vi "GDSProject_Create.vi"(1 "ProjectTreePosition(String or Project Item Ref)":variant, 2 "AllowPopUpDilaog(True)":bool=TRUE, 5 "error in (no error)":errorcluster) -> (14 "Project Refnum":refnum<vi>, 15 "Project Item":refnum<vi>, 17 "App":refnum<vi>, 19 "error out":errorcluster)   [LabVIEW 2016]
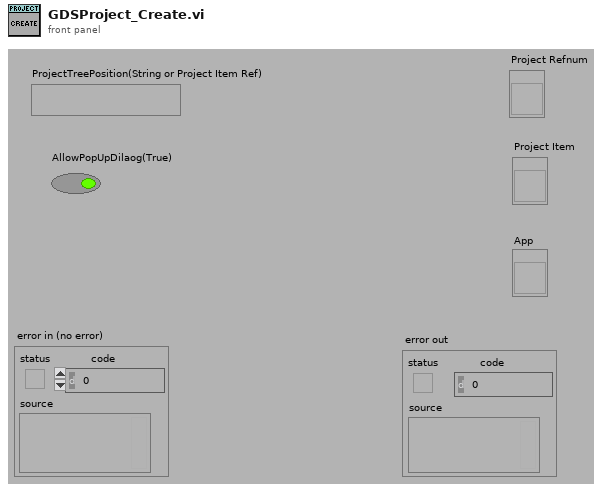
[diagram p1: front panel]
types:
  T1 = enum16{"Left Button", "Center Button", "Right Button", "Window Close"}
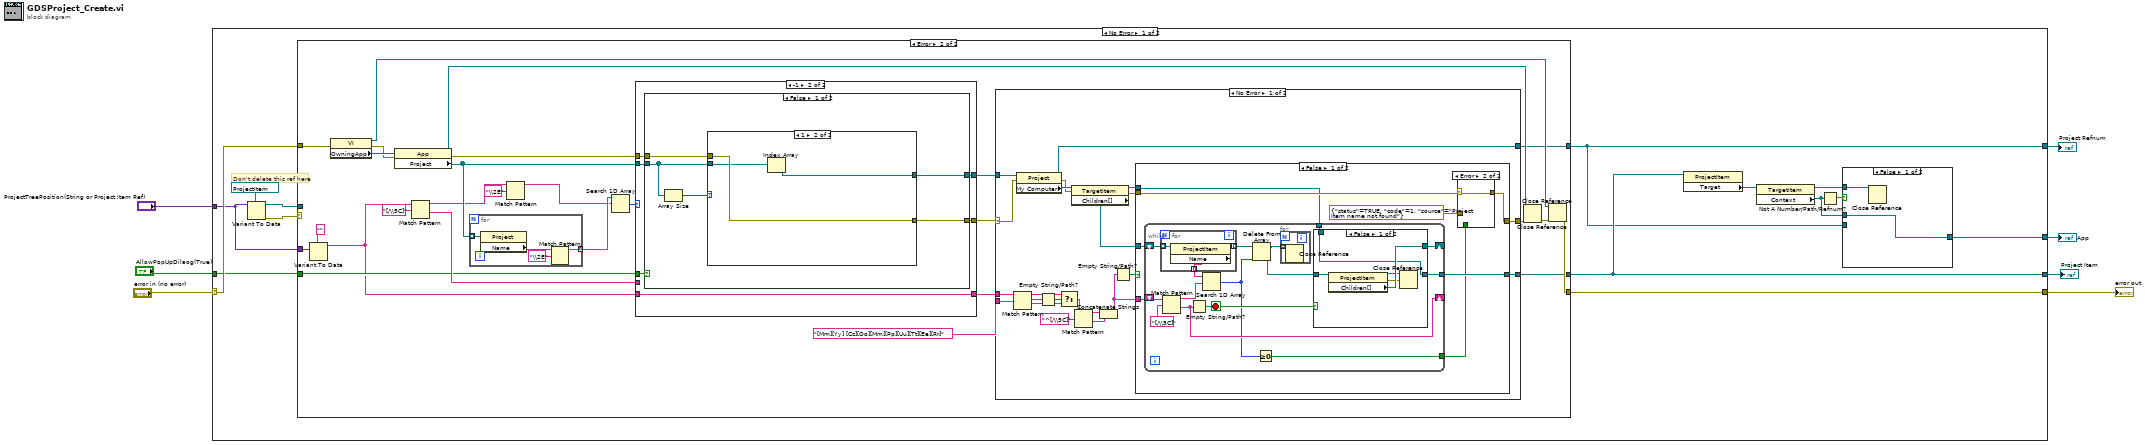
[diagram p0: block diagram]
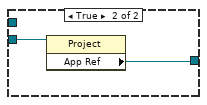
[diagram p2: hidden frame]
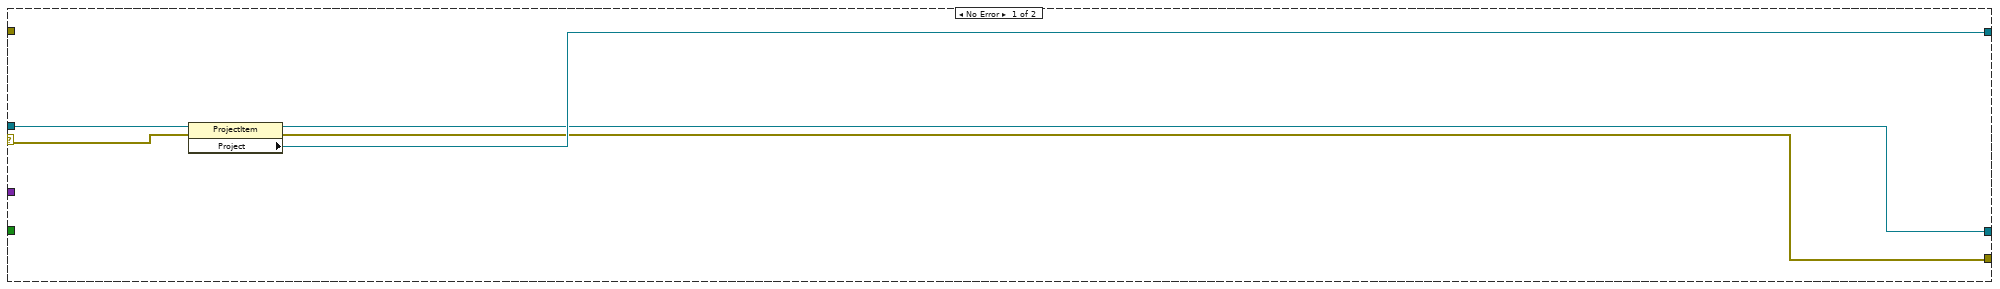
[diagram p3: hidden frame]
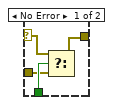
[diagram p4: hidden frame]
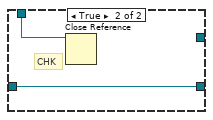
[diagram p5: hidden frame]
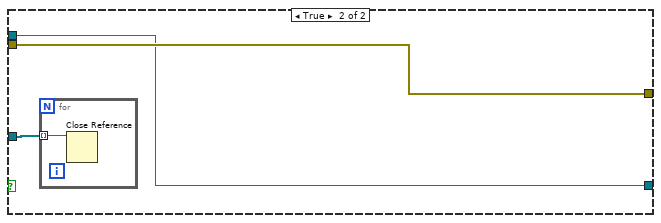
[diagram p6: hidden frame]
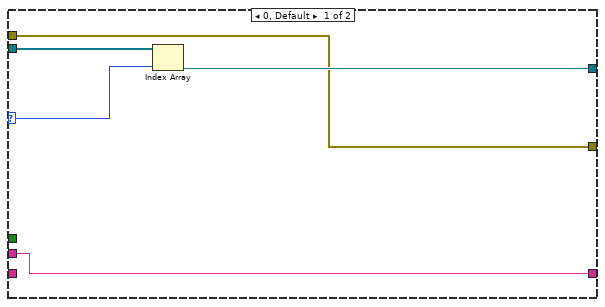
[diagram p8: hidden frame]
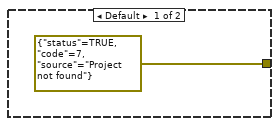
[diagram p9: hidden frame]
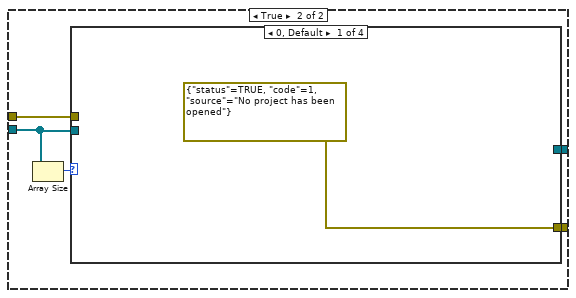
[diagram p10: hidden frame]
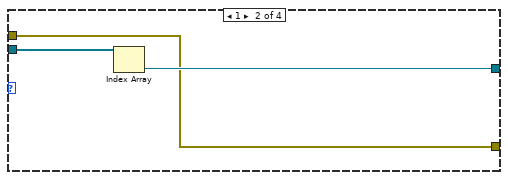
[diagram p11: hidden frame]
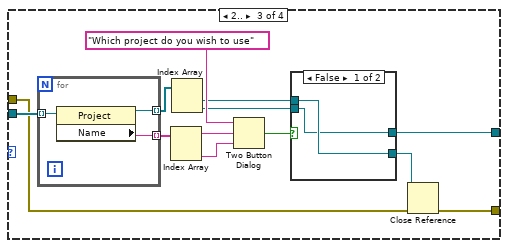
[diagram p12: hidden frame]
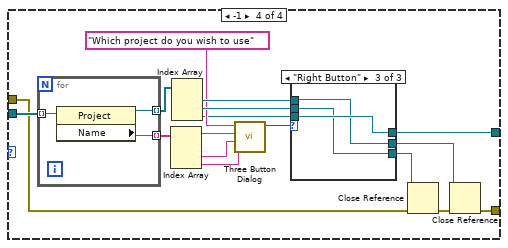
[diagram p14: hidden frame]
diagram:
  n1 = case shown="No Error" "error in (no error)" {
    selector: "error in (no error)" -> [w21 w206]
    tunnel: [w20 w206] -> w6
    tunnel: "ProjectTreePosition(String or Project Item Ref)" -> [w15 _]
    tunnel: [w11 _] -> w4
    tunnel: [w10 _] -> w3
    tunnel: "AllowPopUpDilaog(True)" -> [w19 _]
    tunnel: [w9 _] -> w1
    frame No Error {
      # "Don't delete this ref here"
      n2 = Variant To Data(type=refnum<vi> refnum ("Project Item"), Variant=w15) -> (data=w16:refnum<vi>, error out=w17:errorcluster)  [unwired: 1 in]
      n3 = case shown="Error" w17 {
        selector: w17 -> [w26 _]
        tunnel: w21 -> [_ w56]
        tunnel: [w29 w51] -> w20
        tunnel: [w28 w41] -> w11
        tunnel: [w30 w36] -> w10
        tunnel: w19 -> [_ w35]
        tunnel: w16 -> [w27 _]
        tunnel: w15 -> [_ w33]
        frame No Error {
          n4 = property class="ProjectItem"(reference=w27, error in=w26) -> (reference out=w28:refnum<vi>, error out=w29:errorcluster, "Project"=w30:refnum<vi>)
        }
        frame Error {
          n5 = Variant To Data(type="" ("regular expression"), Variant=w33) -> (data=w31:string)  [unwired: 1 in, 1 out]
          n6 = property class="VI"(error in=w56) -> (reference out=w50:refnum<vi>, error out=w55:errorcluster, "OwningApp"=w57:refnum<vi>)  [unwired: 1 in]
          n7 = property class="App"(reference=w57, error in=w55) -> (reference out=w53:refnum<vi>, error out=w54:errorcluster, "Project"=w49:refnum<vi>[])
          n8 = Match Pattern(string=w31, regular expression="[/\\5C]") -> (before substring=w38:string, after substring=w45:string)  [unwired: 1 in, 2 out]
          n9 = for {
            tunnel: w49 -> [w205] mode=indexing
            tunnel: [w202] -> w47 mode=indexing
            n10 = property class="Project"(reference=w205) -> ("Name"=w203:string)  [unwired: 1 in, 2 out]
            n11 = Match Pattern(string=w203, regular expression="\\2E") -> (before substring=w202:string)  [unwired: 1 in, 3 out]
          }
          n12 = Match Pattern(string=w38, regular expression="\\2E") -> (before substring=w37:string)  [unwired: 1 in, 3 out]
          n13 = Search 1D Array(1D array=w47, element=w37) -> (index of element=w46:i32)  [unwired: 1 in]
          n14 = case shown="-1" w46 {
            selector: w46 -> [w127 _]
            tunnel: [w126 w134] -> w44
            tunnel: w54 -> [w125 w133]
            tunnel: [w125 w132] -> w34
            tunnel: w49 -> [w128 w131]
            tunnel: w31 -> [_ w130]
            tunnel: w45 -> [w124 _]
            tunnel: [w124 w130] -> w43
            tunnel: w35 -> [_ w129]
            frame 0, Default {
              n15 = Index Array(array=w128, index=w127) -> (element=w126:refnum<vi>)
            }
            frame -1 {
              n16 = case shown="False" w129 {
                tunnel: [w135 w148] -> w134
                tunnel: w133 -> [w137 w146]
                tunnel: [w139 w145] -> w132
                tunnel: w131 -> [w136 w144]
                frame False {
                  n17 = Array Size(array=w136) -> (size(s)=w138:i32)
                  n18 = case shown="1" w138 {
                    tunnel: [errorcluster {"status"=TRUE, "code"=7, "source"="Project not found"} ("error out") w143] -> w139
                    tunnel: w137 -> [_ w143]
                    tunnel: w136 -> [_ w142]
                    tunnel: [_ w141] -> w135
                    frame Default {
                    }
                    frame 1 {
                      n19 = Index Array(array=w142) -> (element=w141:refnum<vi>)  [unwired: 1 in]
                    }
                  }
                }
                frame True {
                  n20 = Array Size(array=w144) -> (size(s)=w147:i32)
                  n21 = case shown="0, Default" w147 {
                    tunnel: w144 -> [_ w152 w165 w189]
                    tunnel: [_ w151 w157 w185] -> w148
                    tunnel: w146 -> [_ w150 w155 w183]
                    tunnel: [errorcluster {"status"=TRUE, "code"=1, "source"="No project has been opened"} ("error out") w150 w154 w175] -> w145
                    frame 0, Default {
                    }
                    frame 1 {
                      n22 = Index Array(array=w152) -> (element=w151:refnum<vi>)  [unwired: 1 in]
                    }
                    frame 2.. {
                      n23 = for {
                        tunnel: w165 -> [w172] mode=indexing
                        tunnel: [w171] -> w163 mode=indexing
                        tunnel: [w170] -> w160 mode=indexing
                        n24 = property class="Project"(reference=w172) -> (reference out=w170:refnum<vi>, "Name"=w171:string)  [unwired: 1 in, 1 out]
                      }
                      n25 = Index Array(array=w163) -> (element #1=w162:string, element #2=w161:string)  [unwired: 2 in]
                      n26 = Index Array(array=w160) -> (element #1=w158:refnum<vi>, element #2=w156:refnum<vi>)  [unwired: 2 in]
                      n27 = Two Button Dialog(message="Which project do you wish to use", 1:w161, 2:w162) -> (T button?=w159:bool)
                      n28 = case shown="False" w159 {
                        tunnel: w158 -> [w167 w169]
                        tunnel: [w166 w169] -> w157
                        tunnel: [w167 w168] -> w153
                        tunnel: w156 -> [w166 w168]
                        frame False {
                        }
                        frame True {
                        }
                      }
                      n29 = Close Reference(reference=w153, error in (no error)=w155) -> (error out=w154:errorcluster)
                    }
                    frame -1 {
                      n30 = for {
                        tunnel: w189 -> [w201] mode=indexing
                        tunnel: [w200] -> w188 mode=indexing
                        tunnel: [w199] -> w187 mode=indexing
                        n31 = property class="Project"(reference=w201) -> (reference out=w199:refnum<vi>, "Name"=w200:string)  [unwired: 1 in, 1 out]
                      }
                      n32 = Index Array(array=w188) -> (element #1=w180:string, element #2=w179:string, element #3=w178:string)  [unwired: 3 in]
                      n33 = Index Array(array=w187) -> (element #1=w186:refnum<vi>, element #2=w184:refnum<vi>, element #3=w174:refnum<vi>)  [unwired: 3 in]
                      n34 = call <vilib>:"Three Button Dialog.vi"("Right Button Text (\"Cancel\")"=w178, "Center Button Text (\"No\")"=w179, "Left Button Text (\"Yes\")"=w180, "message"="Which project do you wish to use") -> ("Which Button?"=w177:T1)  [unwired: 7 in]
                      n35 = case shown="\"Right Button\"" w177 {
                        tunnel: w186 -> [w192 w194 w197]
                        tunnel: [w192 w195 w198] -> w185
                        tunnel: [w191 w193 w196] -> w182
                        tunnel: w184 -> [w190 w195 w196]
                        tunnel: w174 -> [w191 w193 w198]
                        tunnel: [w190 w194 w197] -> w173
                        frame "Left Button", Default {
                        }
                        frame "Center Button" {
                        }
                        frame "Right Button" {
                        }
                      }
                      n36 = Close Reference(reference=w182, error in (no error)=w183) -> (error out=w176:errorcluster)
                      n37 = Close Reference(reference=w173, error in (no error)=w176) -> (error out=w175:errorcluster)
                    }
                  }
                }
              }
            }
          }
          n38 = case shown="No Error" w34 {
            selector: w34 -> [w59 w123]
            tunnel: w44 -> [w79 _]
            tunnel: w43 -> [w77 _]
            tunnel: "[Mm][Yy] [Cc][Oo][Mm][Pp][Uu][Tt][Ee][Rr]" ("regular expression") -> [w76 _]
            tunnel: [w70 _] -> w41
            tunnel: [w66 w123] -> w40
            tunnel: [w65 _] -> w36
            frame No Error {
              n39 = Match Pattern(string=w77, regular expression=w76) -> (before substring=w73:string, match substring=w75:string, after substring=w72:string)  [unwired: 1 in, 1 out]
              n40 = property class="Project"(reference=w79, error in=w59) -> (reference out=w65:refnum<vi>, error out=w69:errorcluster, "My Computer"=w78:refnum<vi>)
              n41 = Empty String/Path?(string/path=w75) -> (empty?=w74:bool)
              n42 = Select(t=w73, s=w74, f=w72) -> (s? t:f=w64:string)
              n43 = property class="TargetItem"(reference=w78, error in=w69) -> (reference out=w58:refnum<vi>, error out=w67:errorcluster, "Children[]"=w71:refnum<vi>[])
              n44 = Match Pattern(string=w64, regular expression="^[/\\5C]") -> (before substring=w62:string, after substring=w61:string)  [unwired: 1 in, 2 out]
              n45 = Concatenate Strings(w62, w61) -> (w60:string)
              n46 = Empty String/Path?(string/path=w60) -> (empty?=w68:bool)
              n47 = case shown="False" w68 {
                tunnel: w71 -> [w87 w119]
                tunnel: [w86 w120] -> w70
                tunnel: w60 -> [w85 _]
                tunnel: w67 -> [w84 w121]
                tunnel: [w82 w121] -> w66
                tunnel: w58 -> [w80 w120]
                frame False {
                  n48 = while {
                    shift-right: [w100] -> _
                    shift-left: w87 -> [w107]
                    tunnel: [w99] -> w86
                    shift-right: [w97] -> _
                    shift-left: w85 -> [w98]
                    tunnel: [w95] -> w83
                    tunnel: w80 -> [w93]
                    stop <- w102 stop-if-true
                    n49 = for {
                      tunnel: w107 -> [w118] mode=indexing
                      tunnel: [w117] -> w106 mode=indexing
                      tunnel: [w116] -> w104 mode=indexing
                      n50 = property class="ProjectItem"(reference=w118) -> (reference out=w116:refnum<vi>, "Name"=w117:string)  [unwired: 1 in, 1 out]
                    }
                    n51 = Match Pattern(string=w98, regular expression="[/\\5C]") -> (before substring=w105:string, after substring=w97:string)  [unwired: 1 in, 2 out]
                    n52 = Empty String/Path?(string/path=w97) -> (empty?=w102:bool)
                    n53 = Search 1D Array(1D array=w106, element=w105) -> (index of element=w94:i32)  [unwired: 1 in]
                    n54 = Delete From Array(array=w104, index=w94) -> (deleted portion=w101:refnum<vi>, array with subset deleted=w103:refnum<vi>[])  [unwired: 1 in]
                    n55 = Greater Or Equal To 0?(x=w94) -> (x >= 0?=w95:bool)
                    n56 = for {
                      tunnel: w103 -> [w115] mode=indexing
                      n57 = Close Reference(reference=w115) -> ()  [unwired: 1 in, 1 out]
                    }
                    n58 = case shown="False" w102 {
                      tunnel: w101 -> [w112 w114]
                      tunnel: [w111 _] -> w100
                      tunnel: [w108 w114] -> w99
                      tunnel: w93 -> [w108 w113]
                      frame False {
                        n59 = property class="ProjectItem"(reference=w112) -> (reference out=w109:refnum<vi>, error out=w110:errorcluster, "Children[]"=w111:refnum<vi>[])  [unwired: 1 in]
                        n60 = Close Reference(reference=w109, error in (no error)=w110) -> ()  [unwired: 1 out]
                      }
                      frame True {
                        # "CHK"
                        n61 = Close Reference(reference=w113) -> ()  [unwired: 1 in, 1 out]
                      }
                    }
                  }
                  n62 = case shown="Error" w84 {
                    selector: w84 -> [w90 w92]
                    tunnel: w83 -> [w91 _]
                    tunnel: [w89 w92] -> w82
                    tunnel: errorcluster {"status"=TRUE, "code"=1, "source"="Project Item name not found"} ("f") -> [w88 _]
                    frame No Error {
                      n63 = Select(t=w90, s=w91, f=w88) -> (s? t:f=w89:errorcluster)
                    }
                    frame Error {
                    }
                  }
                }
                frame True {
                  n64 = for {
                    tunnel: w119 -> [w122] mode=indexing
                    n65 = Close Reference(reference=w122) -> ()  [unwired: 1 in, 1 out]
                  }
                }
              }
            }
            frame Error {
            }
          }
          n66 = Close Reference(reference=w53, error in (no error)=w40) -> (error out=w52:errorcluster)
          n67 = Close Reference(reference=w50, error in (no error)=w52) -> (error out=w51:errorcluster)
        }
      }
      n68 = property class="ProjectItem"(reference=w11) -> ("Target"=w14:refnum<vi>)  [unwired: 1 in, 2 out]
      n69 = property class="TargetItem"(reference=w14) -> (reference out=w8:refnum<vi>, "Context"=w12:refnum<vi>)  [unwired: 1 in, 1 out]
      n70 = Not A Number/Path/Refnum?(number/path/refnum=w12) -> (NaN/Path/Refnum?=w13:bool)
      n71 = case shown="False" w13 {
        tunnel: [w23 w25] -> w9
        tunnel: w10 -> [_ w24]
        tunnel: w12 -> [w23 _]
        tunnel: w8 -> [w22 _]
        frame False {
          n72 = Close Reference(reference=w22) -> ()  [unwired: 1 in, 1 out]
        }
        frame True {
          n73 = property class="Project"(reference=w24) -> ("App Ref"=w25:refnum<vi>)  [unwired: 1 in, 2 out]
        }
      }
    }
    frame Error {
    }
  }
  "Project Refnum" <- w3
  "error out" <- w6
  "Project Item" <- w4
  "App" <- w1
